vi "fetch image.vi"(8 "error in (no error)":errorcluster, 11 "MeritFactor in":refnum<class "MeritFactor.lvclass">) -> (0 "error out":errorcluster, 3 "MeritFactor out":refnum<class "MeritFactor.lvclass">)   [LabVIEW 2012, in "MeritFactor.lvclass"]
uses:
  MeritFactor.lvclass
  MeritFactor.lvclass/MeritFactor.ctl
  <vilib>/Distrio/Murmex/FetchMessage/FetchMessage.lvclass
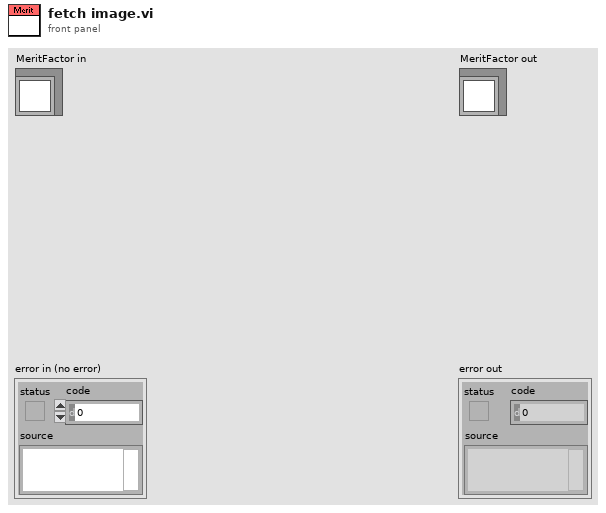
[diagram p1: front panel]
types:
  T1 = typedef "Murmex.lvlib/FetchMessage.lvclass/Channel data cluster.ctl" = cluster{"channel id":i32, "data UInt8":u8[], "data type":T2, "dimensions":i32[], "physical units":T3[], "waveform dt":dbl, "waveform":T4}
  T2 = typedef "Murmex.lvlib/Murmex.lvclass/data_type_enum.ctl" = enum16{"Float128", "Float64", "Float32", "Int64", "Int32", "Int16", "Int8", "UInt64", "UInt32", "UInt16", "UInt8", "Boolean", "String"}
  T3 = typedef "Physical Units__ogtk.ctl" = cluster{"Base Units":enum16{"radian", "steradian", "second", "meter", "kilogram", "ampere", "kelvin", "mole", "candela"}, "Exponent":i16}
  T4 = typedef "Murmex.lvlib/Murmex.lvclass/waveform_type_enum.ctl" = enum16{"no waveform", "analog", "digital"}
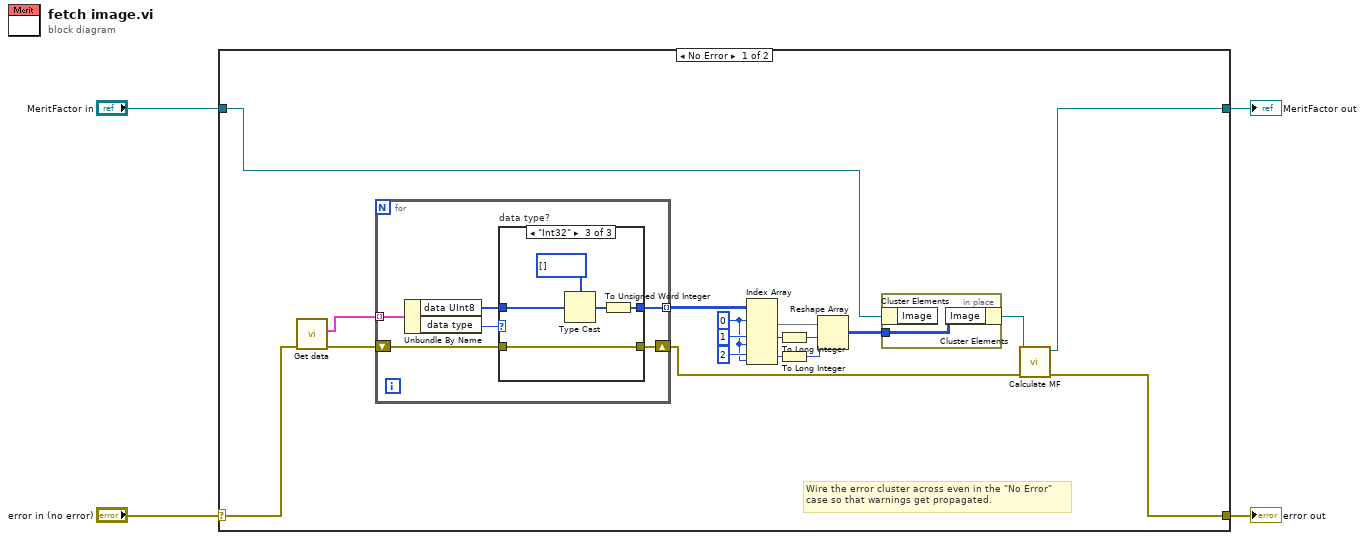
[diagram p0: block diagram]
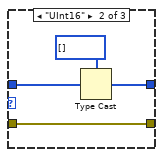
[diagram p3: hidden frame]
diagram:
  n1 = case shown="No Error" "error in (no error)" {
    selector: "error in (no error)" -> [w8 w41]
    tunnel: [w7 w41] -> w3
    tunnel: [w5 w40] -> w1
    tunnel: "MeritFactor in" -> [w6 w40]
    frame No Error {
      w14 = 0 ("index (row)")
      # "Wire the error cluster across even in the \"No Error\"\ncase so that warnings get propagated."
      n2 = call <vilib>:"Get data.vi"("error in (no error)"=w8) -> ("error out"=w22:errorcluster, "data (channels)"=w21:T1[])  [unwired: 8 in, 1 out]
      n3 = for {
        shift-right: [w26] -> w11
        shift-left: w22 -> [w27]
        tunnel: w21 -> [w29] mode=indexing
        tunnel: [w24] -> w20 mode=indexing
        n4 = Unbundle By Name(w29) -> ("data UInt8"=w25:u8[], "data type"=w28:T2)
        n5 = case "data type?" shown="\"Int32\"" w28 {
          tunnel: w27 -> [w30 w34 w36]
          tunnel: [w30 w34 w36] -> w26
          tunnel: w25 -> [_ w33 w39]
          tunnel: [_ w31 w35] -> w24
          frame Default {
          }
          frame "UInt16" {
            n6 = Type Cast(type=u16[] [], x=w33) -> (*(type *) &x=w31:u16[])
          }
          frame "Int32" {
            n7 = Type Cast(type=i32[] [], x=w39) -> (*(type *) &x=w37:i32[])
            n8 = To Unsigned Word Integer(number=w37) -> (unsigned 16bit integer=w35:u16[])
          }
        }
      }
      n9 = Index Array(array=w20, index (row) #1=w14, index (row) #2=1 ("index (col)"), index (col) #2=w14, index (row) #3=2 ("index (row)"), index (col) #3=w14) -> (element #1=w18:u16[], element #2=w17:u16, element #3=w12:u16)  [unwired: 1 in]
      n10 = To Long Integer(number=w17) -> (32bit integer=w16:i32)
      n11 = To Long Integer(number=w12) -> (32bit integer=w13:i32)
      n12 = Reshape Array(w18, w16, w13) -> (w9:u16[][])
      n13 = in-place {
        in-place-border: w9 -> [w23]
        n14 = in-place-cluster #1(w6) -> ()  [unwired: 1 out]
        n15 = in-place-cluster #1("Image"=w23) -> (w10:refnum<class "MeritFactor.lvclass">)
      }
      n16 = call-dynamic "Calculate MF.vi"("error in (no error)"=w11, "MeritFactor in"=w10) -> ("error out"=w7:errorcluster, "MeritFactor out"=w5:refnum<class "MeritFactor.lvclass">)  [unwired: 8 in]
    }
    frame Error {
    }
  }
  "error out" <- w3
  "MeritFactor out" <- w1
